vi "Relay Map.vi"(4 "Relay":T1) -> (1 "bit":u8)   [LabVIEW 2012]
uses:
  Relay Name.ctl
panel:
  in  "Map":u8[](array[numeric])=[6, 7, 5, 3, 2, 1, 0, 4]
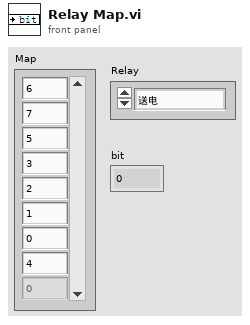
[diagram p1: front panel]
types:
  T1 = typedef "Relay Name.ctl" = enum8{"送电", "液压站", "润滑电机", "冷却电机", "滑台快进", "滑台工进", "滑台快退", "报警指示灯"}
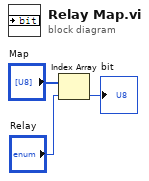
[diagram p0: block diagram]
diagram:
  n1 = Index Array(array="Map", index="Relay") -> (element=→"bit":u8)
